vi "PRIME Detector Format Command.vi"(11 "Command":string="STATUS") -> (3 "TCP String":string)   [LabVIEW 2024, in "PRIME Detector.lvclass"]
uses:
  PRIME Detector.lvclass
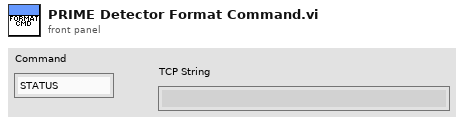
[diagram p1: front panel]
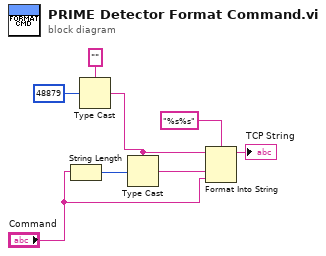
[diagram p0: block diagram]
diagram:
  n1 = String Length(string="Command") -> (length=w4:i32)
  n2 = Type Cast(type="", x=u16 48879) -> (*(type *) &x=w3:string)
  n3 = Type Cast(type=w3, x=w4) -> (*(type *) &x=w2:string)
  n4 = Format Into String(format string="%s%s", initial string=w3, w2, "Command") -> (resulting string=→"TCP String":string)  [unwired: 1 in, 1 out]
